vi "3-4.vi"() -> ()   [LabVIEW 2018]
panel:
  out "Waveform Chart":dynamicdata(graph)
  out "number (0 to 1)":dbl
  in  "stop":bool
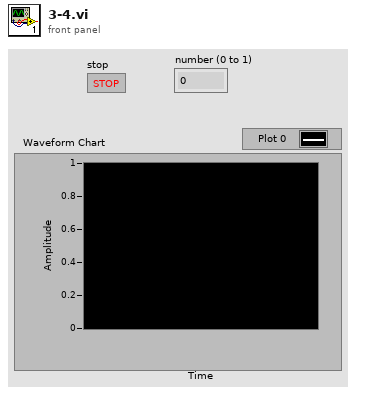
[diagram p1: front panel]
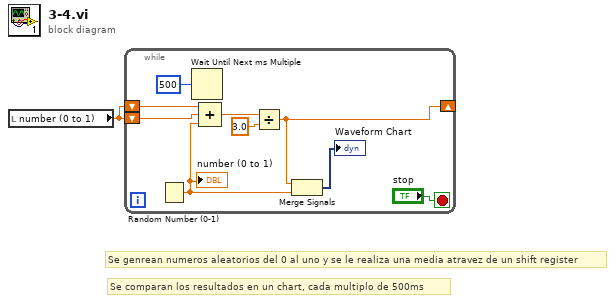
[diagram p0: block diagram]
diagram:
  # "Se comparan los resultados en un chart, cada multiplo de 500ms"
  # "Se genrean numeros aleatorios del 0 al uno y se le realiza una media atravez de un shift register"
  n1 = local read "number (0 to 1)"() -> (w1:dbl)
  n2 = while {
    shift-right: [w6] -> _
    shift-left: w1 -> [w5]
    shift-left: w1 -> [w4]
    stop <- "stop" stop-if-true
    n3 = Random Number (0-1)() -> (number: 0 to 1=w3:dbl)
    "number (0 to 1)" <- w3
    n4 = Wait Until Next ms Multiple(millisecond multiple=u32 500) -> ()  [unwired: 1 out]
    n5 = Compound Arithmetic op=ADD(w5, w4, w3) -> (w10:dbl)
    n6 = Divide(x=w10, y=3.0) -> (x/y=w6:dbl)
    n7 = Merge Signals(w6, w3) -> (→"Waveform Chart":dynamicdata)
  }
